vi "ACK_Control.vi"(8 "error in (no error)":errorcluster, 9 "Producer In":T1={"Temps(K)"=[], "Fields(T)"=[], "Sweep States"=enum."1. Idle", "PointStep"=enum."1. Scan_1", "Current Field"=0.0, "Current Temp"=0.0, "Expected_ACK"=enum."1. None", "ACK"=enum."1. None", "AfterAckStep"=enum."1. Idle", "Current Index Field"=0, "Current Index Temp"=0, "ACK Structure "=enum."Inner"}, 10 "ACK Q":refnum<queue>, 11 "Queue in":refnum<queue>) -> (0 "error out":errorcluster, 2 "Producer out":T1={"Temps(K)"=[], "Fields(T)"=[], "Sweep States"=enum."1. Idle", "PointStep"=enum."1. Scan_1", "Current Field"=0.0, "Current Temp"=0.0, "Expected_ACK"=enum."1. None", "ACK"=enum."1. None", "AfterAckStep"=enum."1. Idle", "Current Index Field"=0, "Current Index Temp"=0, "ACK Structure "=enum."Inner"}, 3 "Queue out":refnum<queue>)   [LabVIEW 2025]
uses:
  CTLS/Sweeper.ctl
  CTLS/ACK.ctl
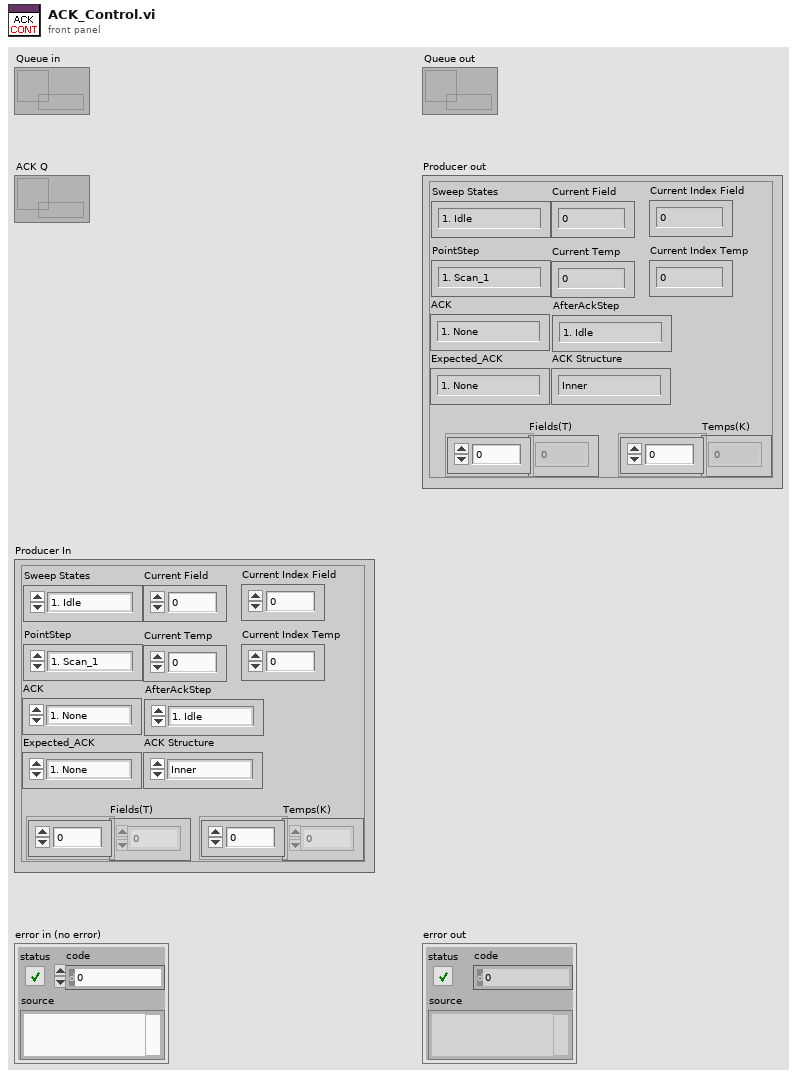
[diagram p1: front panel]
types:
  T1 = typedef "Sweeper.ctl" = cluster{"Temps(K)":dbl[], "Fields(T)":dbl[], "Sweep States":enum16{"1. Idle", "2. Start", "3. Apply_Config", "4. Run_Point_Step", "5. Wait ACK", "6. Next Field", "7. Next Temp", "8. Stop"}, "PointStep":enum16{"1. Init_Bias", "2. Init_Scan", "3. Field_Stable", "4. Temp_stable", "1. Scan_1", "2. DC_SF_1", "3. DC_BS_1", "4. Bias", "5. Scan_2", "6. DC_SF_2", "7. DC_BS_2", "8. Done"}, "Current Field":dbl, "Current Temp":dbl, "Expected_ACK":enum16{"1. None", "2. TempStable", "3. FieldStable", "4. ConfigApplied", "5. ScanDone", "6. BiasDone", "7. DriftDone (SF)", "8. DrifDone (BS)", "9. Done"}, "ACK":enum16{"1. None", "2. TempStable", "3. FieldStable", "4. ConfigApplied", "5. ScanDone", "6. BiasDone", "7. DriftDone (SF)", "8. DrifDone (BS)", "9. Done"}, "AfterAckStep":enum16{"1. Idle", "2. Start", "3. Apply_Config", "4. Run_Point_Step", "5. Wait ACK", "6. Next Field", "7. Next Temp", "8. Stop"}, "Current Index Field":i32, "Current Index Temp":i32, "ACK Structure ":enum16{"Inner", "Outer"}}
  T2 = typedef "ACK.ctl" = cluster{"ACK":enum16{"1. None", "2. TempStable", "3. FieldStable", "4. ConfigApplied", "5. ScanDone", "6. BiasDone", "7. DriftDone (SF)", "8. DrifDone (BS)"}}
  T3 = enum16{"1. None", "2. TempStable", "3. FieldStable", "4. ConfigApplied", "5. ScanDone", "6. BiasDone", "7. DriftDone (SF)", "8. DrifDone (BS)", "9. Done"}
  T4 = enum16{"1. None", "2. TempStable", "3. FieldStable", "4. ConfigApplied", "5. ScanDone", "6. BiasDone", "7. DriftDone (SF)", "8. DrifDone (BS)"}
  T5 = enum16{"1. Idle", "2. Start", "3. Apply_Config", "4. Run_Point_Step", "5. Wait ACK", "6. Next Field", "7. Next Temp", "8. Stop"}
  T6 = enum16{"1. Init_Bias", "2. Init_Scan", "3. Field_Stable", "4. Temp_stable", "1. Scan_1", "2. DC_SF_1", "3. DC_BS_1", "4. Bias", "5. Scan_2", "6. DC_SF_2", "7. DC_BS_2", "8. Done"}
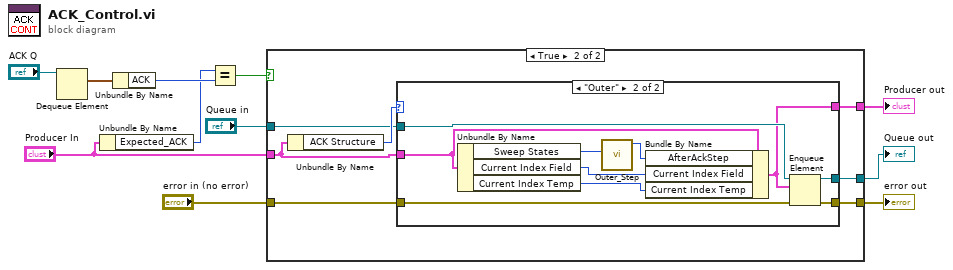
[diagram p0: block diagram]
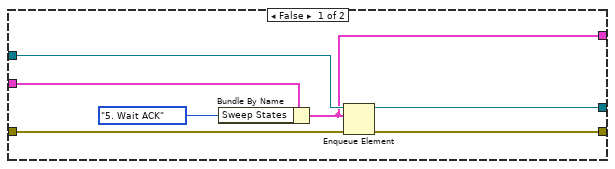
[diagram p2: hidden frame]
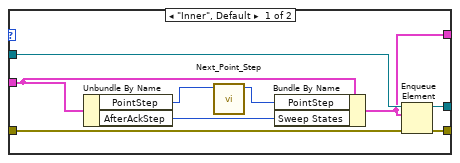
[diagram p3: hidden frame]
diagram:
  n1 = Dequeue Element(queue="ACK Q") -> (element=w2:T2)  [unwired: 2 in, 3 out]
  n2 = Unbundle By Name("Producer In") -> ("Expected_ACK"=w3:T3)
  n3 = Unbundle By Name(w2) -> ("ACK"=w4:T4)
  n4 = Equal?(x=w3, y=w4) -> (x = y?=w5:bool)
  n5 = case shown="True" w5 {
    tunnel: "Queue in" -> [w18 w23]
    tunnel: "Producer In" -> [w17 w19]
    tunnel: [w16 w22] -> w8
    tunnel: [w15 w21] -> w9
    tunnel: "error in (no error)" -> [w14 w20]
    tunnel: [w13 w24] -> w11
    frame False {
      n6 = Bundle By Name(cluster=w17, "Sweep States"=T5."5. Wait ACK") -> (w13:T1)
      n7 = Enqueue Element(queue=w18, element=w13, error in (no error)=w14) -> (queue out=w16:refnum<queue>, error out=w15:errorcluster)  [unwired: 1 in, 1 out]
    }
    frame True {
      n8 = Unbundle By Name(w19) -> ("ACK Structure"=w25:enum16{"Inner", "Outer"})
      n9 = case shown="\"Outer\"" w25 {
        tunnel: w19 -> [w29 w40]
        tunnel: [w30 w39] -> w24
        tunnel: w23 -> [w34 w44]
        tunnel: [w33 w43] -> w22
        tunnel: [w32 w42] -> w21
        tunnel: w20 -> [w31 w41]
        frame "Inner", Default {
          n10 = Unbundle By Name(w29) -> ("PointStep"=w27:T6, "AfterAckStep"=w28:T5)
          n11 = call "Next_Point_Step.vi"("Current State"=w27) -> ("Next State"=w26:T6)  [unwired: 10 in]
          n12 = Bundle By Name(cluster=w29, "PointStep"=w26, "Sweep States"=w28) -> (w30:T1)
          n13 = Enqueue Element(queue=w34, element=w30, error in (no error)=w31) -> (queue out=w33:refnum<queue>, error out=w32:errorcluster)  [unwired: 1 in, 1 out]
        }
        frame "Outer" {
          n14 = Unbundle By Name(w40) -> ("Sweep States"=w38:T5, "Current Index Field"=w36:i32, "Current Index Temp"=w35:i32)
          n15 = call "Outer_Step.vi"("Sweep States"=w38) -> ("AfterAckStep out"=w37:T5)  [unwired: 10 in]
          n16 = Bundle By Name(cluster=w40, "AfterAckStep"=w37, "Current Index Field"=w36, "Current Index Temp"=w35) -> (w39:T1)
          n17 = Enqueue Element(queue=w44, element=w39, error in (no error)=w41) -> (queue out=w43:refnum<queue>, error out=w42:errorcluster)  [unwired: 1 in, 1 out]
        }
      }
    }
  }
  "Producer out" <- w11
  "error out" <- w9
  "Queue out" <- w8
